vi "倒计时器.vi"() -> ()   [LabVIEW 2017]
panel:
  out "?":bool
  out "倒计时":string
  in  "停止":bool
  in  "开始倒计时":bool
  in  "定时时间选择":enum16{"6秒", "10秒", "20秒"}(ring)
  # "倒 计 时 器"
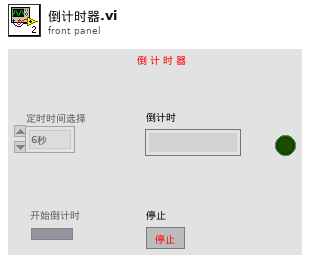
[diagram p1: front panel]
types:
  T1 = enum8{"Enabled", "Disabled", "Disabled and Grayed Out"}
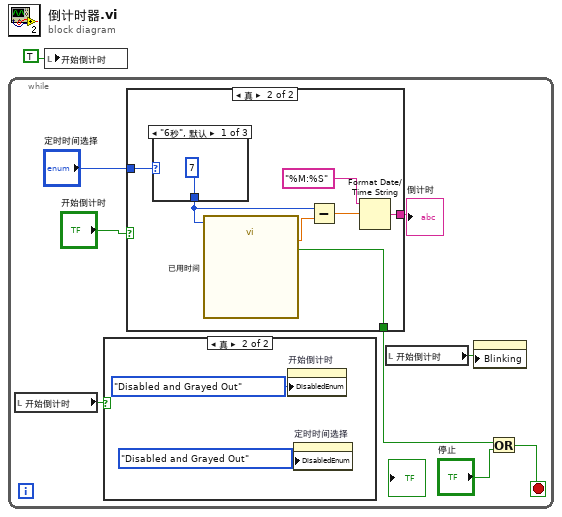
[diagram p0: block diagram]
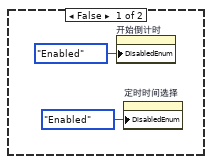
[diagram p2: hidden frame]
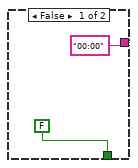
[diagram p3: hidden frame]
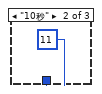
[diagram p4: hidden frame]
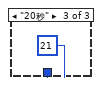
[diagram p5: hidden frame]
diagram:
  n1 = while {
    stop <- w2 stop-if-true
    n2 = local read "开始倒计时"() -> (w5:bool)
    n3 = case shown="真" w5 {
      frame False {
        n4 = property on="开始倒计时" class="Bool (严格)"("DisabledEnum"=T1."Enabled" ("禁用")) -> ()  [unwired: 2 in, 2 out]
        n5 = property on="定时时间选择" class="Enum (严格)"("DisabledEnum"=T1."Enabled" ("禁用")) -> ()  [unwired: 2 in, 2 out]
      }
      frame True {
        n6 = property on="开始倒计时" class="Bool (严格)"("DisabledEnum"=T1."Disabled and Grayed Out" ("禁用")) -> ()  [unwired: 2 in, 2 out]
        n7 = property on="定时时间选择" class="Enum (严格)"("DisabledEnum"=T1."Disabled and Grayed Out" ("禁用")) -> ()  [unwired: 2 in, 2 out]
      }
    }
    n8 = case shown="真" "开始倒计时" {
      tunnel: "定时时间选择" -> [_ w22]
      tunnel: [FALSE w16] -> w3
      tunnel: ["00:00" ("date/time string") w17] -> w7
      frame False {
      }
      frame True {
        n9 = case shown="\"6秒\", 默认" w22 {
          tunnel: [7 11 21] -> w21
          frame "6秒", Default {
          }
          frame "10秒" {
          }
          frame "20秒" {
          }
        }
        n10 = call "已用时间"("Time Target (s)"=w21) -> ("Elapsed Time (s)"=w20:dbl, "Time has Elapsed"=w16:bool)  [unwired: 11 in, 6 out]
        n11 = Subtract(x=w21, y=w20) -> (x-y=w19:dbl)
        n12 = Format Date/Time String(time format string (%c)="%M:%S" ("时间格式字符串(%c)"), seconds (now)=w19) -> (date/time string=w17:string)  [unwired: 1 in]
      }
    }
    "倒计时" <- w7
    n13 = local read "开始倒计时"() -> (w9:bool)
    n14 = property class="Bool (严格)"("Blinking"=w9) -> ()  [unwired: 2 in, 2 out]
    n15 = Or(x=w3, y="停止") -> (x .or. y?=w2:bool)
  }
  n16 = local write "开始倒计时"(TRUE) -> ()
